vi "模拟温度测量.vi"() -> ()   [LabVIEW 2014]
panel:
  in  "采集的电压\n（传感器输出）":dbl
  out "温度值":dbl
  in  "温度单位\n（上 C 下 F）":bool
  out "温度计":dbl(slide) scale=0.0..100.0
  # "摄氏度 C"
  # "华氏度 F"
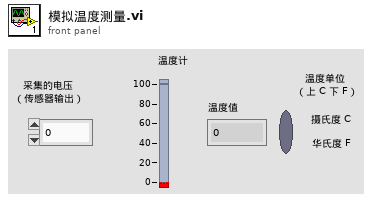
[diagram p1: front panel]
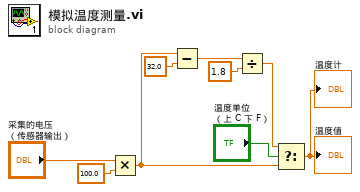
[diagram p0: block diagram]
diagram:
  n1 = Multiply(x="采集的电压\n（传感器输出）", y=100.0) -> (x*y=w3:dbl)
  n2 = Subtract(x=w3, y=32.0) -> (x-y=w6:dbl)
  n3 = Divide(x=w6, y=1.8) -> (x/y=w2:dbl)
  n4 = Select(t=w2, s="温度单位\n（上 C 下 F）", f=w3) -> (s? t:f=→"温度计" →"温度值":dbl)
